vi "New Run Trigger.vi"(8 "error in":errorcluster, 11 "CaptureDetectionLoopDataIn":T1={"Period"=-1, "Reset"=TRUE, "Trigger"=FALSE, "Iteration"=0, "Capture"=path "", "Mode"=enum."Record", "Replay Run ID"="", "Module Launched Timestamp"=timestamp(0 s since 1904-01-01)}) -> (0 "error out":errorcluster, 2 "Trigger":bool, 3 "CaptureDetectionLoopDataOut":T1={"Period"=-1, "Reset"=TRUE, "Trigger"=FALSE, "Iteration"=0, "Capture"=path "", "Mode"=enum."Record", "Replay Run ID"="", "Module Launched Timestamp"=timestamp(0 s since 1904-01-01)})   [LabVIEW 2026, in "Launcher.lvlib"]
uses:
  Launcher.lvlib
  Capture detection loop data--cluster.ctl
  Mode.ctl
  082daf70-e610-4a57-b030-8ff7e5508b21.vi
  <userlib>/_OpenG.lib/file/file.llb/openg_file.lvlib
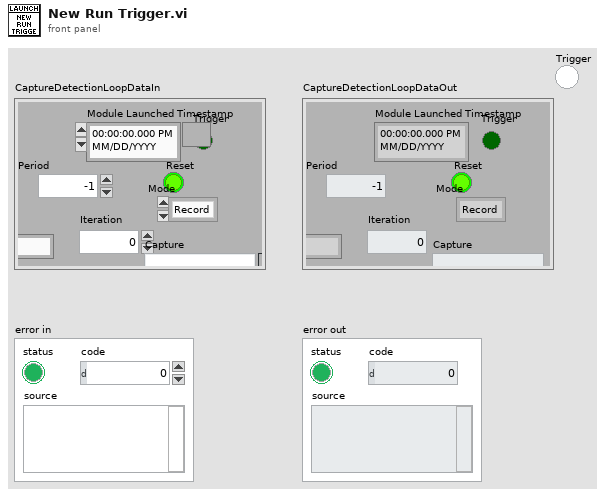
[diagram p1: front panel]
types:
  T1 = typedef "Capture detection loop data--cluster.ctl" = cluster{"Period":i32, "Reset":bool, "Trigger":bool, "Iteration":i32, "Capture":path, "Mode":T2, "Replay Run ID":string, "Module Launched Timestamp":timestamp}
  T2 = typedef "Mode.ctl" = enum16{"Record", "Record and Replay"}
  T3 = typedef "openg_file.lvlib/File Info Record__ogtk.ctl" = cluster{"type":string, "creator":string, "permissions":i32, "data size":i32, "res size":i32, "creation date":u32, "modification date":u32, "bFolder":bool, "bInvisible":bool, "location":cluster{"vertical":i16, "horizontal":i16}, "owner":string, "group":string}
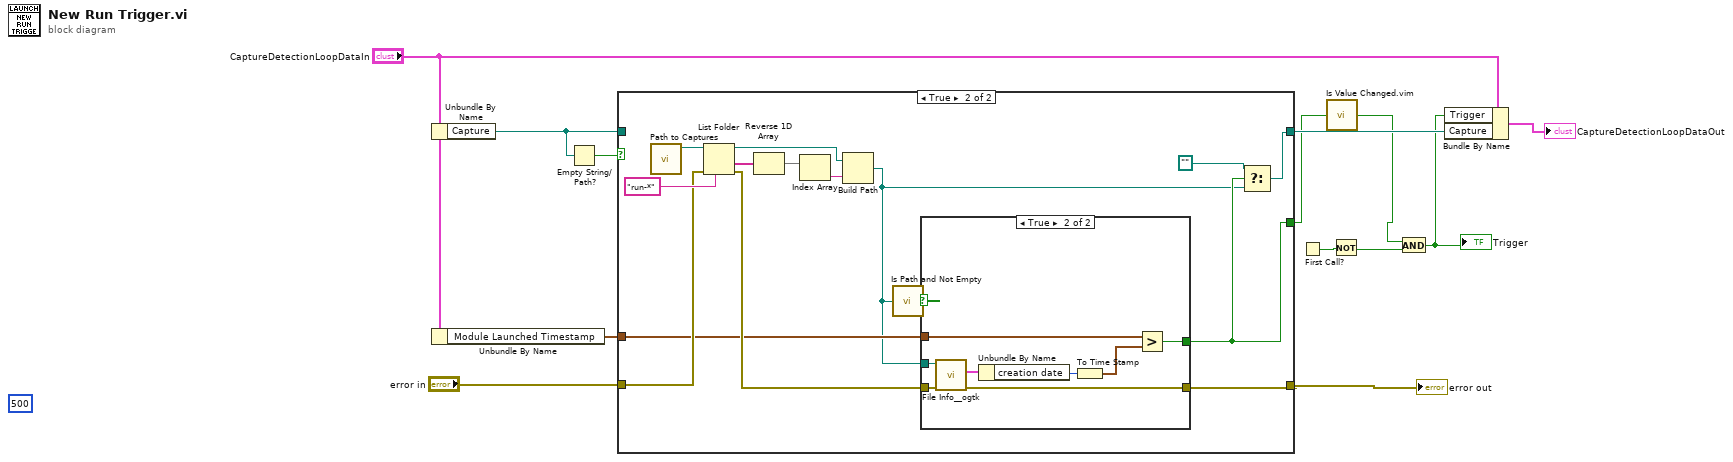
[diagram p0: block diagram]
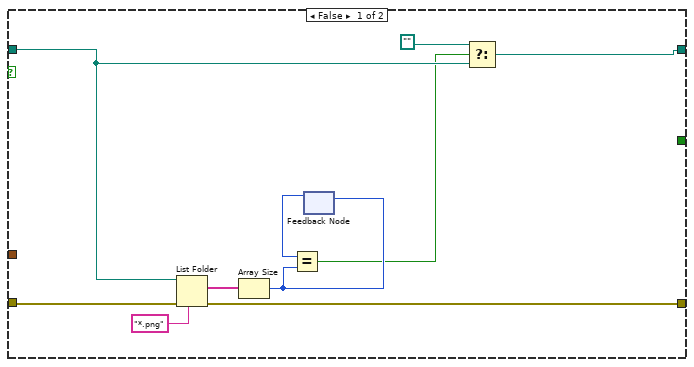
[diagram p2: hidden frame]
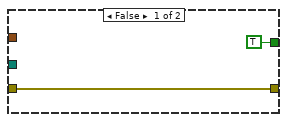
[diagram p3: hidden frame]
diagram:
  (unwired) 500
  n1 = Unbundle By Name("CaptureDetectionLoopDataIn") -> ("Capture"=w8:path)
  n2 = Unbundle By Name("CaptureDetectionLoopDataIn") -> ("Module Launched Timestamp"=w6:timestamp)
  n3 = Empty String/Path?(string/path=w8) -> (empty?=w9:bool)
  n4 = case shown="True" w9 {
    tunnel: "error in" -> [w23 w33]
    tunnel: [_ w26] -> w5
    tunnel: [w16 w27] -> w10
    tunnel: w8 -> [w17 _]
    tunnel: [w14 w30] -> w11
    tunnel: w6 -> [_ w29]
    frame False {
      n5 = List Folder(path=w17, pattern="*.png", error in=w23) -> (filenames=w21:string[], error out=w14:errorcluster)  [unwired: 1 in, 2 out]
      n6 = Array Size(array=w21) -> (size(s)=w20:i32)
      n7 = feedback-in #1(w20) -> ()
      n8 = feedback #1() -> (w19:i32)  [unwired: 1 in]
      n9 = Equal?(x=w19, y=w20) -> (x = y?=w15:bool)
      n10 = Select(t=path "", s=w15, f=w17) -> (s? t:f=w16:path)
    }
    frame True {
      n11 = call "Path to Captures.vi"() -> ("Captures"=w32:path)  [unwired: 11 in]
      n12 = List Folder(path=w32, pattern="run-*", error in=w33) -> (path out=w34:path, folder names=w38:string[], error out=w31:errorcluster)  [unwired: 1 in, 1 out]
      n13 = Reverse 1D Array(array=w38) -> (reversed array=w37:string[])
      n14 = Index Array(array=w37) -> (element=w36:string)  [unwired: 1 in]
      n15 = Build Path(base path=w34, name or relative path=w36) -> (appended path=w25:path)
      n16 = call <vilib>:"Is Path and Not Empty.vi"("path"=w25) -> ("Is Path and Not Empty?"=w24:bool)  [unwired: 4 in]
      n17 = case shown="True" w24 {
        tunnel: w31 -> [w40 w48]
        tunnel: [w40 w46] -> w30
        tunnel: w29 -> [_ w44]
        tunnel: [TRUE w42] -> w26
        tunnel: w25 -> [_ w41]
        frame False {
        }
        frame True {
          n18 = call <userlib>:"File Info__ogtk.vi"("error in (no error)"=w48, "file"=w41) -> ("error out"=w46:errorcluster, "file info"=w47:T3)  [unwired: 4 in, 1 out]
          n19 = Unbundle By Name(w47) -> ("creation date"=w45:u32)
          n20 = To Time Stamp(1:w45) -> (0:w43:timestamp)
          n21 = Greater?(x=w44, y=w43) -> (0:w42:bool)
        }
      }
      n22 = Select(t=path "", s=w26, f=w25) -> (s? t:f=w27:path)
    }
  }
  "error out" <- w11
  n23 = First Call?() -> (First Call?: T/F=w4:bool)
  n24 = call "Is Value Changed.vim"("value"=w5) -> ("changed or first call?"=w2:bool)
  n25 = Not(x=w4) -> (.not. x?=w3:bool)
  n26 = And(x=w2, y=w3) -> (x .and. y?=w1:bool)
  "Trigger" <- w1
  n27 = Bundle By Name(cluster="CaptureDetectionLoopDataIn", "Trigger"=w1, "Capture"=w10) -> (→"CaptureDetectionLoopDataOut":T1)
